vi "U01_12UDPRead.vi"() -> ()   [LabVIEW 2019]
panel:
  out "error out":errorcluster
  out "data out":string
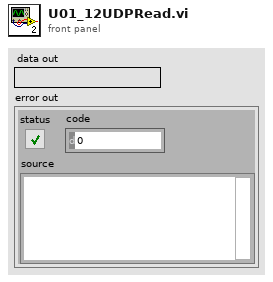
[diagram p1: front panel]
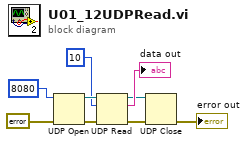
[diagram p0: block diagram]
diagram:
  n1 = UDP Open(8:errorcluster {"status"=FALSE, "code"=0, "source"=""} ("error in (no error)"), 11:u16 8080 ("port")) -> (port=w7:refnum<k16>, 0:w6:errorcluster)  [unwired: 3 in, 1 out]
  n2 = UDP Read(connection ID=w7, max size (548)=10, 8:w6) -> (data out=→"data out":string, error out=w2:errorcluster, 3:w3:refnum<k16>)  [unwired: 1 in, 2 out]
  n3 = UDP Close(connection ID=w3, 8:w2) -> (error out=→"error out":errorcluster)  [unwired: 1 out]
